vi "Correlation_PM1.vi"(0 "shift register D":dbl[](array[numeric])=[0.0, 0.0, 0.0, 0.0, 0.0, 0.0, 0.0, 0.0, 0.0], 2 "Input A":dbl[](array[numeric])=[1.0, 2.0, 5.0, 0.0, 10.0, 1.0, 4.0, 1.0, 2.0], 3 "shift register MY":dbl[](array[numeric])=[0.0, 0.0, 0.0, 0.0, 0.0, 0.0, 0.0, 0.0, 0.0], 5 "m":i32=3, 10 "shift register in":dbl[](array[numeric])=[0.0, 0.0, 0.0, 0.0, 0.0, 0.0, 0.0, 0.0, 0.0], 11 "Acc in":dbl[](array[numeric])=[0.0, 0.0, 0.0, 0.0, 0.0, 0.0, 0.0, 0.0, 0.0]) -> (20 "shift register":dbl[](array[numeric]), 22 "Acc":dbl[](array[numeric]), 23 "shift register Y out":dbl[](array[numeric]), 24 "shift register D out":dbl[](array[numeric]), 25 "MnA":dbl[](array[numeric]))   [LabVIEW 2015]
uses:
  <vilib>/Analysis/NI_AALBase.lvlib
panel:
  out "New Mn":bool=TRUE
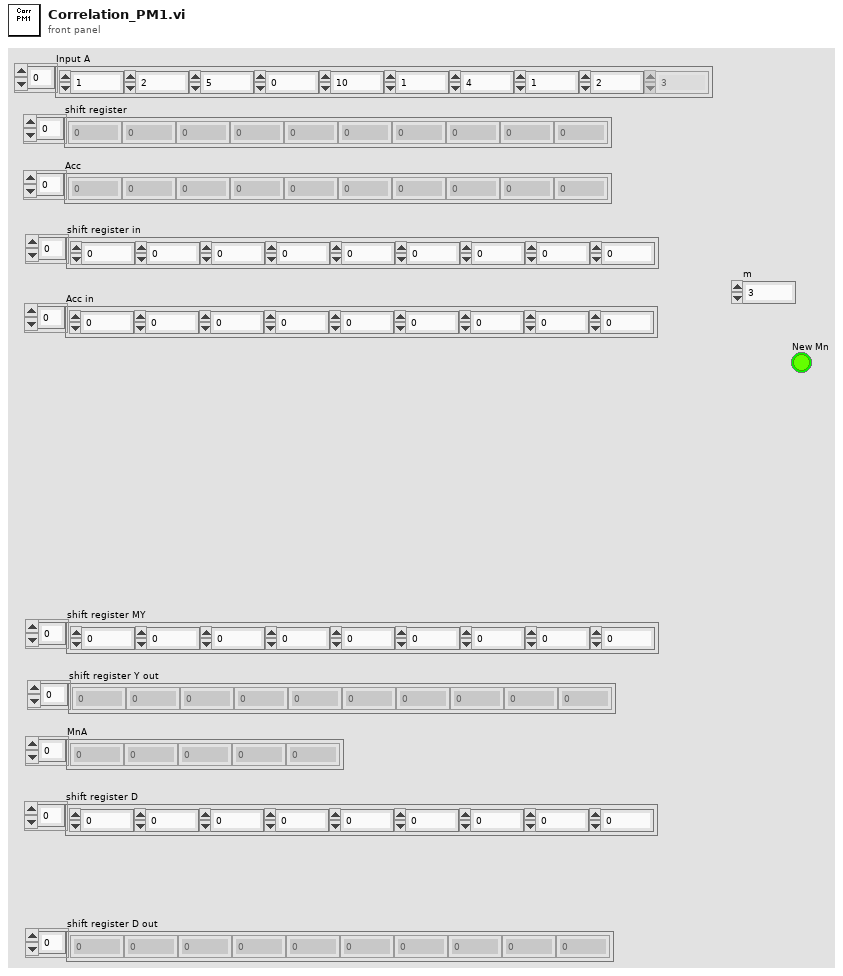
[diagram p1: front panel]
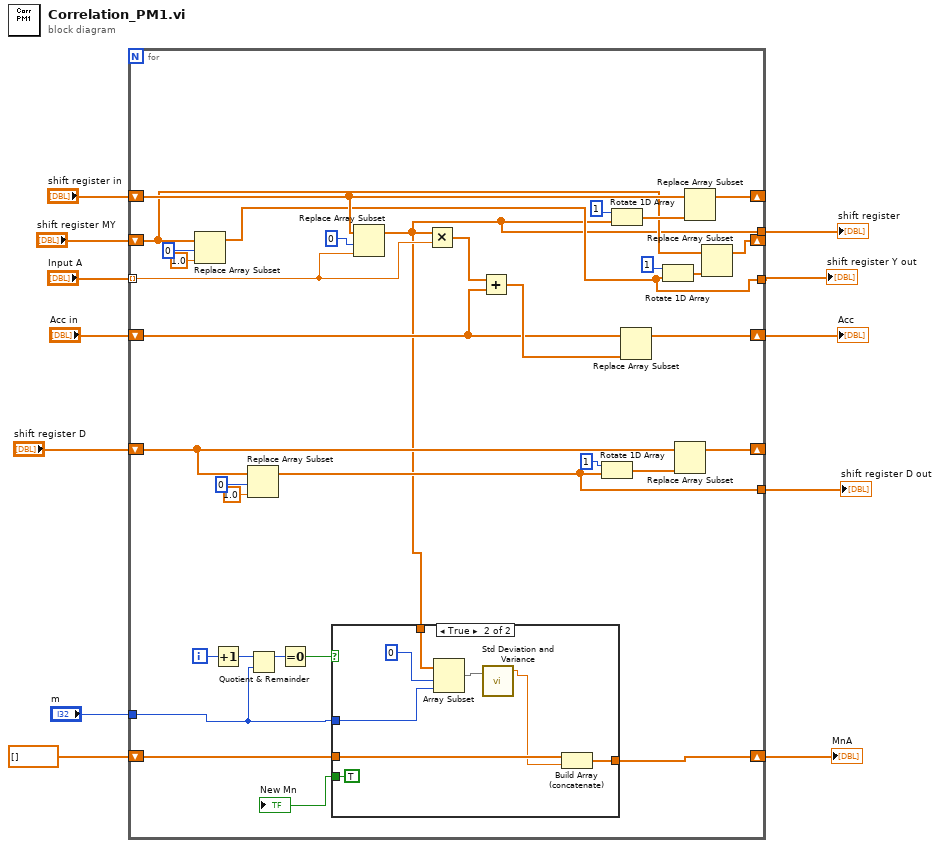
[diagram p0: block diagram]
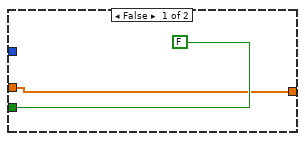
[diagram p2: hidden frame]
diagram:
  n1 = for {
    tunnel: "Input A" -> [w14] mode=indexing
    shift-right: [w41] -> _
    shift-left: "shift register in" -> [w30]
    shift-right: [w39] -> w12
    shift-left: "Acc in" -> [w40]
    tunnel: [w13] -> w11
    shift-right: [w33] -> w7
    shift-left: dbl[] [] -> [w34]
    tunnel: "m" -> [w32]
    shift-right: [w25] -> _
    shift-left: "shift register MY" -> [w24]
    tunnel: [w23] -> w3
    shift-right: [w18] -> _
    shift-left: "shift register D" -> [w16]
    tunnel: [w15] -> w1
    i -> [w22]
    n2 = Replace Array Subset(array=w24, new element=sgl 1.0 ("new element/subarray"), index=0) -> (w23:dbl[])
    n3 = Increment(x=w22) -> (x+1=w37:i32)
    n4 = Replace Array Subset(array=w16, new element=sgl 1.0 ("new element/subarray"), index=0) -> (w15:dbl[])
    n5 = Quotient & Remainder(x=w37, y=w32) -> (x-y*floor(x/y)=w36:i32)  [unwired: 1 out]
    n6 = Equal To 0?(x=w36) -> (x = 0?=w35:bool)
    n7 = Replace Array Subset(array=w30, new element=w14, index=0) -> (w13:dbl[])
    n8 = case shown="True" w35 {
      tunnel: w13 -> [_ w55]
      tunnel: [FALSE TRUE] -> w38
      tunnel: w32 -> [_ w53]
      tunnel: w34 -> [w46 w52]
      tunnel: [w46 w51] -> w33
      frame False {
      }
      frame True {
        n9 = Array Subset(array=w55, index=0, length=w53) -> (w49:dbl[])
        n10 = call <vilib>:"Std Deviation and Variance.vi"("X"=w49) -> ("mean"=w48:dbl)  [unwired: 1 in, 2 out]
        n11 = Build Array (concatenate)(w52, w48) -> (w51:dbl[])
      }
    }
    "New Mn" <- w38
    n12 = Multiply(x=w13, y=w14) -> (x*y=w44:dbl[])
    n13 = Add(x=w44, y=w40) -> (x+y=w43:dbl[])
    n14 = Rotate 1D Array(1:w15, 2:1 ("n")) -> (0:w19:dbl[])
    n15 = Rotate 1D Array(1:w13, 2:1 ("n")) -> (0:w31:dbl[])
    n16 = Replace Array Subset(array=w40, new element=w43) -> (w39:dbl[])  [unwired: 1 in]
    n17 = Rotate 1D Array(1:w23, 2:1 ("n")) -> (0:w26:dbl[])
    n18 = Replace Array Subset(array=w16, new element=w19) -> (w18:dbl[])  [unwired: 1 in]
    n19 = Replace Array Subset(array=w30, new element=w31) -> (w41:dbl[])  [unwired: 1 in]
    n20 = Replace Array Subset(array=w24, new element=w26) -> (w25:dbl[])  [unwired: 1 in]
  }
  "shift register" <- w11
  "Acc" <- w12
  "MnA" <- w7
  "shift register Y out" <- w3
  "shift register D out" <- w1
